vi "Initialize AI.vi"(8 "error in (no error)":errorcluster, 9 "AI Setting":T1={"Physical Channel"=["6363/ai0", "6363/ai1", "6363/ai2"], "Name to assign"=[], "input terminal configuration"=enum."RSE", "minimum value"=0.0, "maximum value"=10.0, "units"=enum."Volts", "custom scale name"="", "sample mode"=enum."Finite Samples", "rate"=5000.0, "samples per channel"=1000} {"rate" format="%#_13g"; "maximum value" format="%#_13g"; "minimum value" format="%#_13g"}, 10 "DAQ Type":enum16{"Hardware", "Simulation"}(ring), 11 "PXIe 6363 in":refnum<class "PXIe 6363.lvclass">) -> (0 "error out":errorcluster, 3 "PXIe 6363 out":refnum<class "PXIe 6363.lvclass">)   [LabVIEW 2021, in "DAQ Hardware.lvlib" / "PXIe 6363.lvclass"]
uses:
  PXIe 6363.lvclass
  User Interface/AI Channel Setting.ctl
  PXIe 6363.lvclass/PXIe 6363.ctl
  DAQ Hardware.lvlib
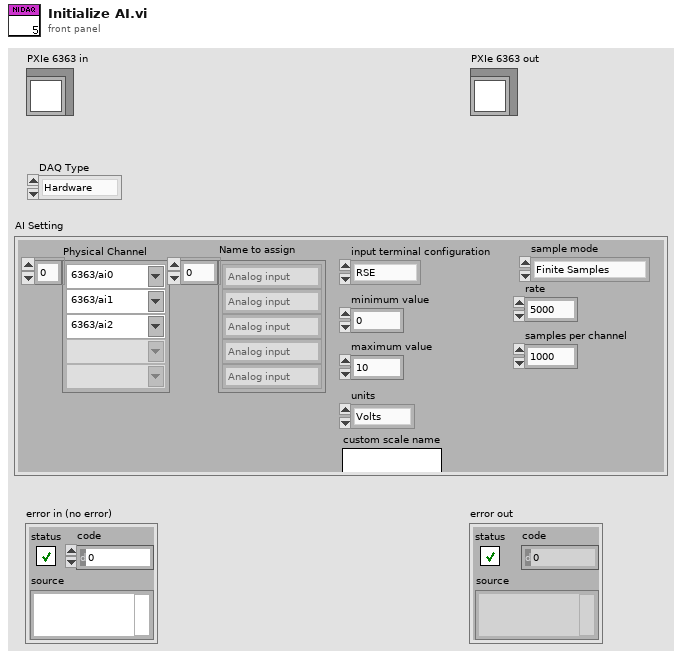
[diagram p1: front panel]
types:
  T1 = typedef "DAQ Hardware.lvlib/AI Channel Setting.ctl" = cluster{"Physical Channel":string[], "Name to assign":string[], "input terminal configuration":enum16{"RSE", "NRSE", "Differential"}, "minimum value":dbl, "maximum value":dbl, "units":enum16{"Volts"}, "custom scale name":string, "sample mode":enum16{"Finite Samples", "Continuous Samples", "Hardware Timed Single Point"}, "rate":dbl, "samples per channel":i32}
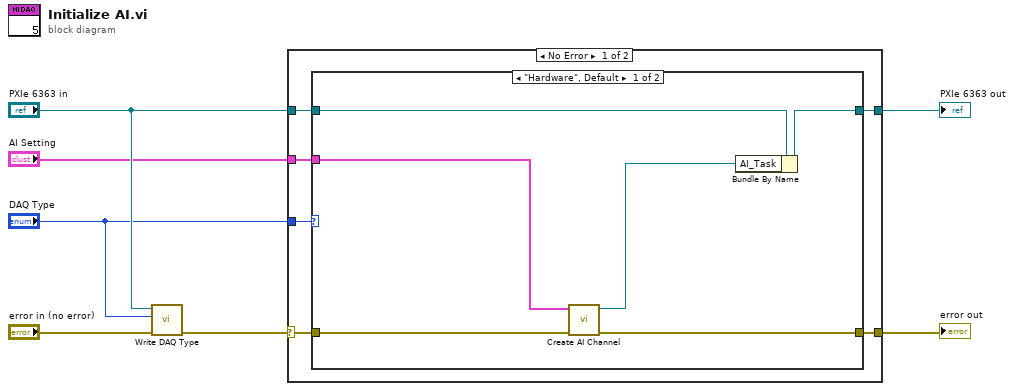
[diagram p0: block diagram]
diagram:
  n1 = call-dynamic "Write DAQ Type.vi"("error in (no error)"="error in (no error)", "DAQ Type"="DAQ Type", "PXIe 6363 in"="PXIe 6363 in") -> ("error out"=w6:errorcluster)  [unwired: 7 in, 1 out]
  n2 = case shown="No Error" w6 {
    selector: w6 -> [w12 w22]
    tunnel: "PXIe 6363 in" -> [w10 w23]
    tunnel: "DAQ Type" -> [w13 _]
    tunnel: [w11 w22] -> w3
    tunnel: [w9 w23] -> w2
    tunnel: "AI Setting" -> [w8 _]
    frame No Error {
      n3 = case shown="\"Hardware\", Default" w13 {
        tunnel: w12 -> [w19 w20]
        tunnel: [w18 w20] -> w11
        tunnel: w10 -> [w14 w21]
        tunnel: [w17 w21] -> w9
        tunnel: w8 -> [w15 _]
        frame "Hardware", Default {
          n4 = call "Create AI Channel.vi"("error in (no error)"=w19, "AI Setting"=w15) -> ("error out"=w18:errorcluster, "task out"=w16:refnum<k21>)  [unwired: 8 in]
          n5 = Bundle By Name(cluster=w14, "AI_Task"=w16) -> (w17:refnum<class "PXIe 6363.lvclass">)
        }
        frame "Simulation" {
        }
      }
    }
    frame Error {
    }
  }
  "error out" <- w3
  "PXIe 6363 out" <- w2
